vi "Convert SequenceFileType.vi"(10 "TSS":T1, 11 "API":i32(ring) items=["SeqFileType_Normal", "SeqFileType_Model", "SeqFileType_FrontEndCBacks", "SeqFileType_StationCBacks", "SeqFileType_Template"]) -> (2 "TSS -> API":i32(ring) items=["SeqFileType_Normal", "SeqFileType_Model", "SeqFileType_FrontEndCBacks", "SeqFileType_StationCBacks", "SeqFileType_Template"], 3 "API -> TSS":T1)   [LabVIEW 2020, in "TSS.lvlib"]
uses:
  TSS.lvlib
  Data Types/Sequence File Type.ctl
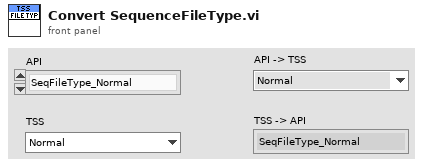
[diagram p1: front panel]
types:
  T1 = typedef "TSS.lvlib/Sequence File Type.ctl" = enum16{"Normal", "Model", "Front End Callbacks", "Station Callbacks", "Template"}
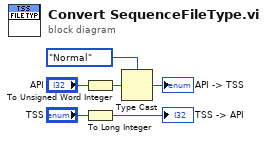
[diagram p0: block diagram]
diagram:
  n1 = To Unsigned Word Integer(number="API") -> (unsigned 16bit integer=w5:u16)
  n2 = To Long Integer(number="TSS") -> (32bit integer=→"TSS -> API":i32)
  n3 = Type Cast(type=Sequence_File_Type."Normal" ("TS -> LV"), x=w5) -> (*(type *) &x=→"API -> TSS":T1)
